vi "Hex to ASCII (SubVI).vi"(11 "Hexadecimal Input String":string="03") -> (3 "String":string)   [LabVIEW 2012]
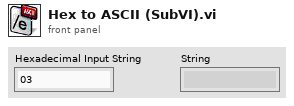
[diagram p1: front panel]
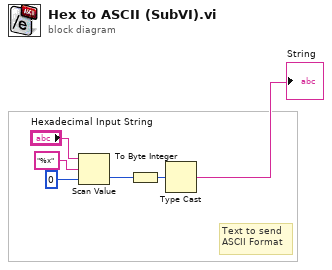
[diagram p0: block diagram]
diagram:
  # "Text to send\nASCII Format"
  n1 = Scan Value(string="Hexadecimal Input String", format string="%x", default (0 dbl)=0) -> (value=w4:i32)  [unwired: 1 out]
  n2 = To Byte Integer(number=w4) -> (8bit integer=w5:i8)
  n3 = Type Cast(x=w5) -> (*(type *) &x=→"String":string)  [unwired: 1 in]
